vi "氨氮通讯.vi"() -> ()   [LabVIEW 2016, in "斯坦道氨氮.lvlib"]
uses:
  <vilib>/NI/Modbus Library/API/Wrapper/Create TCP Slave.vi
  <vilib>/Utility/config.llb/Write Key (String).vi
  <vilib>/Plasmionique/MB Master/MB_Master/MB_Master.lvclass
  <vilib>/NI/Modbus Library/API/slave/Modbus Slave.lvclass
  <vilib>/Utility/config.llb/NI_LVConfig.lvlib
  <vilib>/Plasmionique/MB Master/MB Master.lvlib
  <vilib>/NI/Modbus Library/API/Wrapper/API Main.lvlib
panel:
  out "测量数据区":T1 {"单位" items=["ug/L", "mg/L", "ppm", "mg/m3", "cm", "ppb", "ug/m3", "%", "nmol/mol", "umol/mol", "MPN/L", "MPN/100ml", "ng/m3", "NTU", "无量纲", "ms/cm", "us/cm", "℃", "mV", "万个/L"]}
  out "状态告警区":u16[](array[numeric])
  out "测量数据区":u16[](array[numeric])
  out "序列号":string
  out "状态告警区":T2
  out "status":bool
  out "关键参数区":T3
  in  "读关键参数区":bool
  in  "读状态告警区":bool
  in  "读测量数据区":bool
  in  "站号":u16(ring) items=["总磷"=1, "氨氮"=3]
  in  "停止":bool
  in  "启动":bool
  in  "控制命令":u16(ring) items=["启动测量"=1, "标样核查"=2, "零点核查"=3, "跨度核查"=4, "空白测试"=5, "平行样测试"=6, "加标回收"=7, "空白校准"=8, "标样校准"=9, "初始化（清洗）"=10, "停止测试"=11, "仪器重启"=12, "校时"=13, "模式设置"=14, "测量间隔设置"=15]
  in  "控制命令参数":u16[](array[numeric]) format="%04xH"
  in  "VISA Resource":refnum<visa-resource-name>
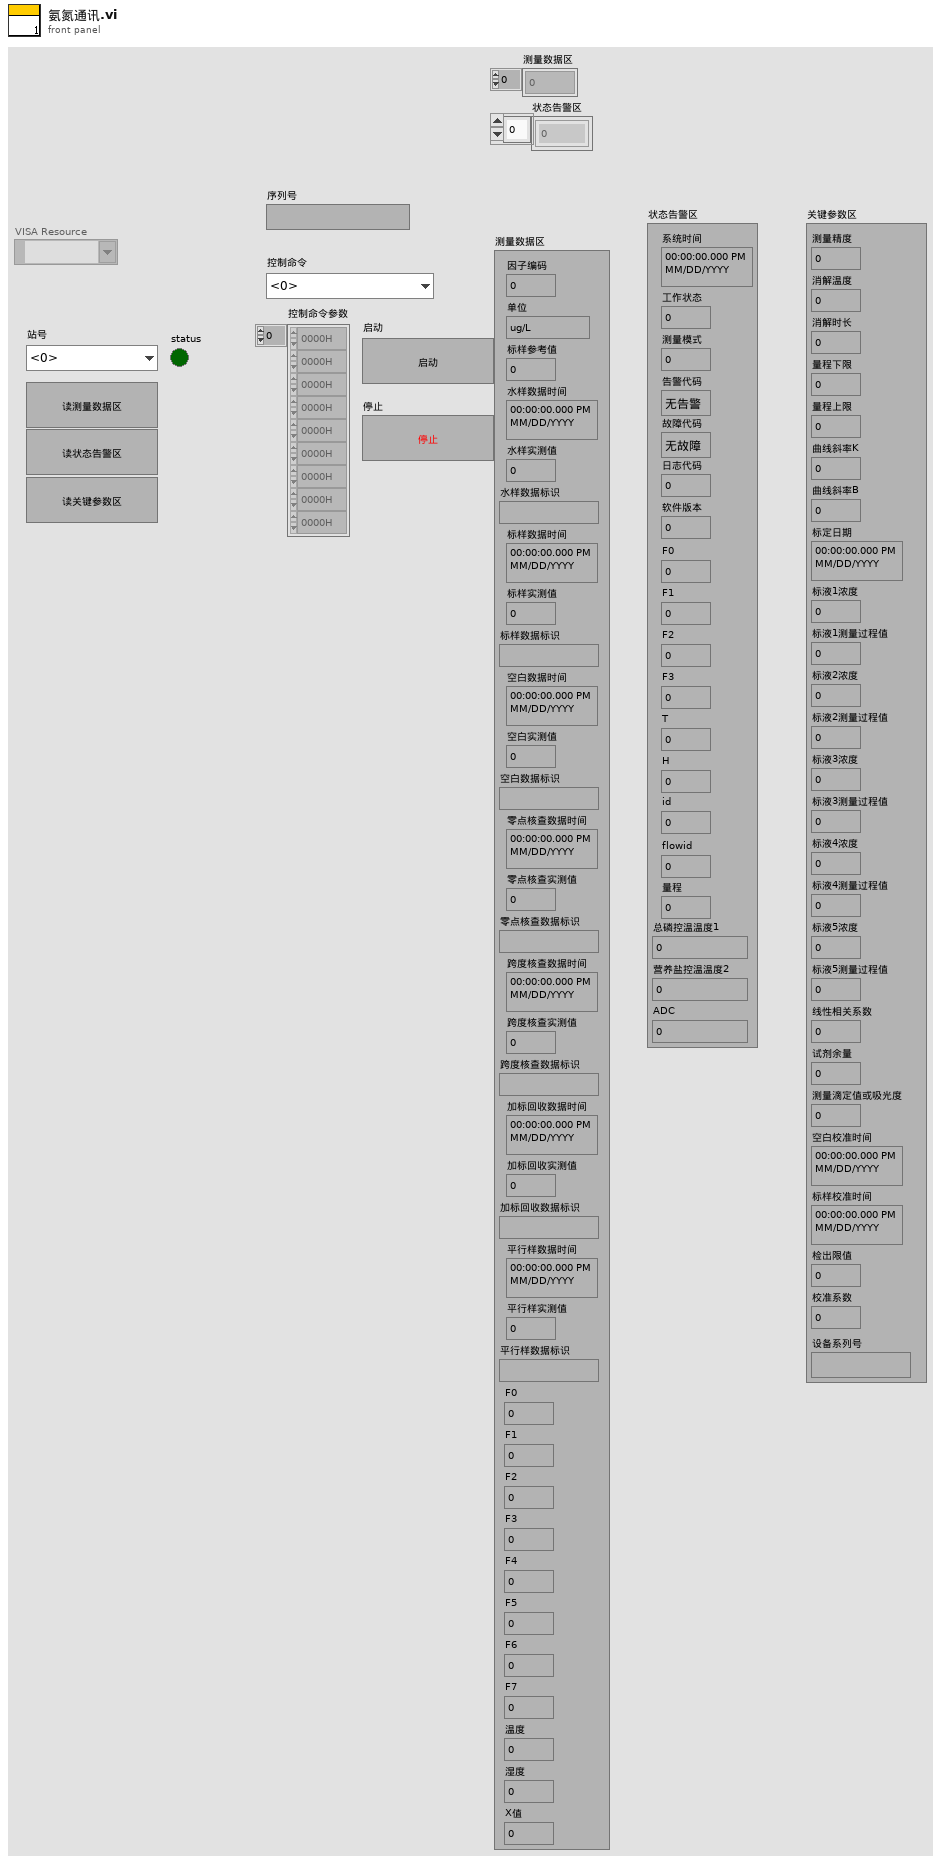
[diagram p1: front panel]
types:
  T1 = cluster{"因子编码":u32, "单位":u16, "标样参考值":sgl, "水样数据时间":timestamp, "水样实测值":sgl, "水样数据标识":string, "标样数据时间":timestamp, "标样实测值":sgl, "标样数据标识":string, "空白数据时间":timestamp, "空白实测值":sgl, "空白数据标识":string, "零点核查数据时间":timestamp, "零点核查实测值":sgl, "零点核查数据标识":string, "跨度核查数据时间":timestamp, "跨度核查实测值":sgl, "跨度核查数据标识":string, "加标回收数据时间":timestamp, "加标回收实测值":sgl, "加标回收数据标识":string, "平行样数据时间":timestamp, "平行样实测值":sgl, "平行样数据标识":string, "F0":sgl, "F1":sgl, "F2":sgl, "F3":sgl, "F4":sgl, "F5":sgl, "F6":sgl, "F7":sgl, "温度":sgl, "湿度":sgl, "X值":sgl}
  T2 = cluster{"系统时间":timestamp, "工作状态":u16, "测量模式":u16, "告警代码":enum16{"无告警", "缺试剂告警", "缺水样告警", "缺蒸馏水告警", "缺标液告警", "仪表漏液告警", "标定异常告警", "超量程告警", "加热异常", "低试剂预警", "超上限告警", "超下限告警", "仪表内部其他异常", "滴定异常告警", "电极异常告警", "量程切换告警", "参数设置告警", "PH电极电位异常", "电导率电极异常", "浊度光度异常", "溶解氧电极异常", "溶解氧光强异常", "温度异常告警", "PH异常告警", "溶解氧异常告警", "电导率异常告警", "浊度异常告警", "叶绿素异常告警", "藻密度异常告警", "蓝绿藻异常告警", "ORP异常告警", "氨氮异常告警", "清洁刷异常告警", "SD卡异常告警", "蓝牙异常告警", "Wifi异常告警", "流程异常告警"}, "故障代码":enum16{"无故障", "电机故障", "温度故障", "通讯故障", "滴定故障"}, "日志代码":u16, "软件版本":u16, "F0":sgl, "F1":sgl, "F2":sgl, "F3":sgl, "T":sgl, "H":sgl, "id":u16, "flowid":u16, "量程":u16, "ADC":sgl, "营养盐控温温度2":sgl, "总磷控温温度1":sgl}
  T3 = cluster{"测量精度":u16, "消解温度":u16, "消解时长":u16, "量程下限":sgl, "量程上限":sgl, "曲线斜率K":sgl, "曲线斜率B":sgl, "标定日期":timestamp, "标液1浓度":sgl, "标液1测量过程值":sgl, "标液2浓度":sgl, "标液2测量过程值":sgl, "标液3浓度":sgl, "标液3测量过程值":sgl, "标液4浓度":sgl, "标液4测量过程值":sgl, "标液5浓度":sgl, "标液5测量过程值":sgl, "线性相关系数":sgl, "试剂余量":u32, "测量滴定值或吸光度":sgl, "空白校准时间":timestamp, "标样校准时间":timestamp, "检出限值":sgl, "校准系数":sgl, "设备系列号":string}
  T4 = typedef "NI_LVConfig.lvlib/Config Data RefNum.ctl" = refnum<k1>
  T5 = enum8{"Enabled", "Disabled", "Disabled and Grayed Out"}
  T6 = cluster{"系统时间":timestamp, "工作状态":enum16{"空闲", "水样测试", "标样核查", "零点核查", "跨度核查", "空白测试", "平行样测试", "加标回收", "空白校准", "标样校准", "初始化（清洗）"}, "测量模式":enum16{"待机", "连续模式", "周期模式", "定点模式", "受控模式", "手动模式"}, "告警代码":enum16{"无告警", "缺试剂告警", "缺水样告警", "缺蒸馏水告警", "缺标液告警", "仪表漏液告警", "标定异常告警", "超量程告警", "加热异常", "低试剂预警", "超上限告警", "超下限告警", "仪表内部其他异常", "滴定异常告警", "电极异常告警", "量程切换告警", "参数设置告警", "PH电极电位异常", "电导率电极异常", "浊度光度异常", "溶解氧电极异常", "溶解氧光强异常", "温度异常告警", "PH异常告警", "溶解氧异常告警", "电导率异常告警", "浊度异常告警", "叶绿素异常告警", "藻密度异常告警", "蓝绿藻异常告警", "ORP异常告警", "氨氮异常告警", "清洁刷异常告警", "SD卡异常告警", "蓝牙异常告警", "Wifi异常告警", "流程异常告警"}, "故障代码":enum16{"无故障", "电机故障", "温度故障", "通讯故障", "滴定故障"}, "日志代码":u16, "软件版本":u16, "F0":sgl, "F1":sgl, "F2":sgl, "F3":sgl, "T":sgl, "H":sgl, "id":u16, "flowid":u16, "量程":u16, "总磷控温温度1":sgl, "营养盐控温温度2":sgl, "ADC":sgl}
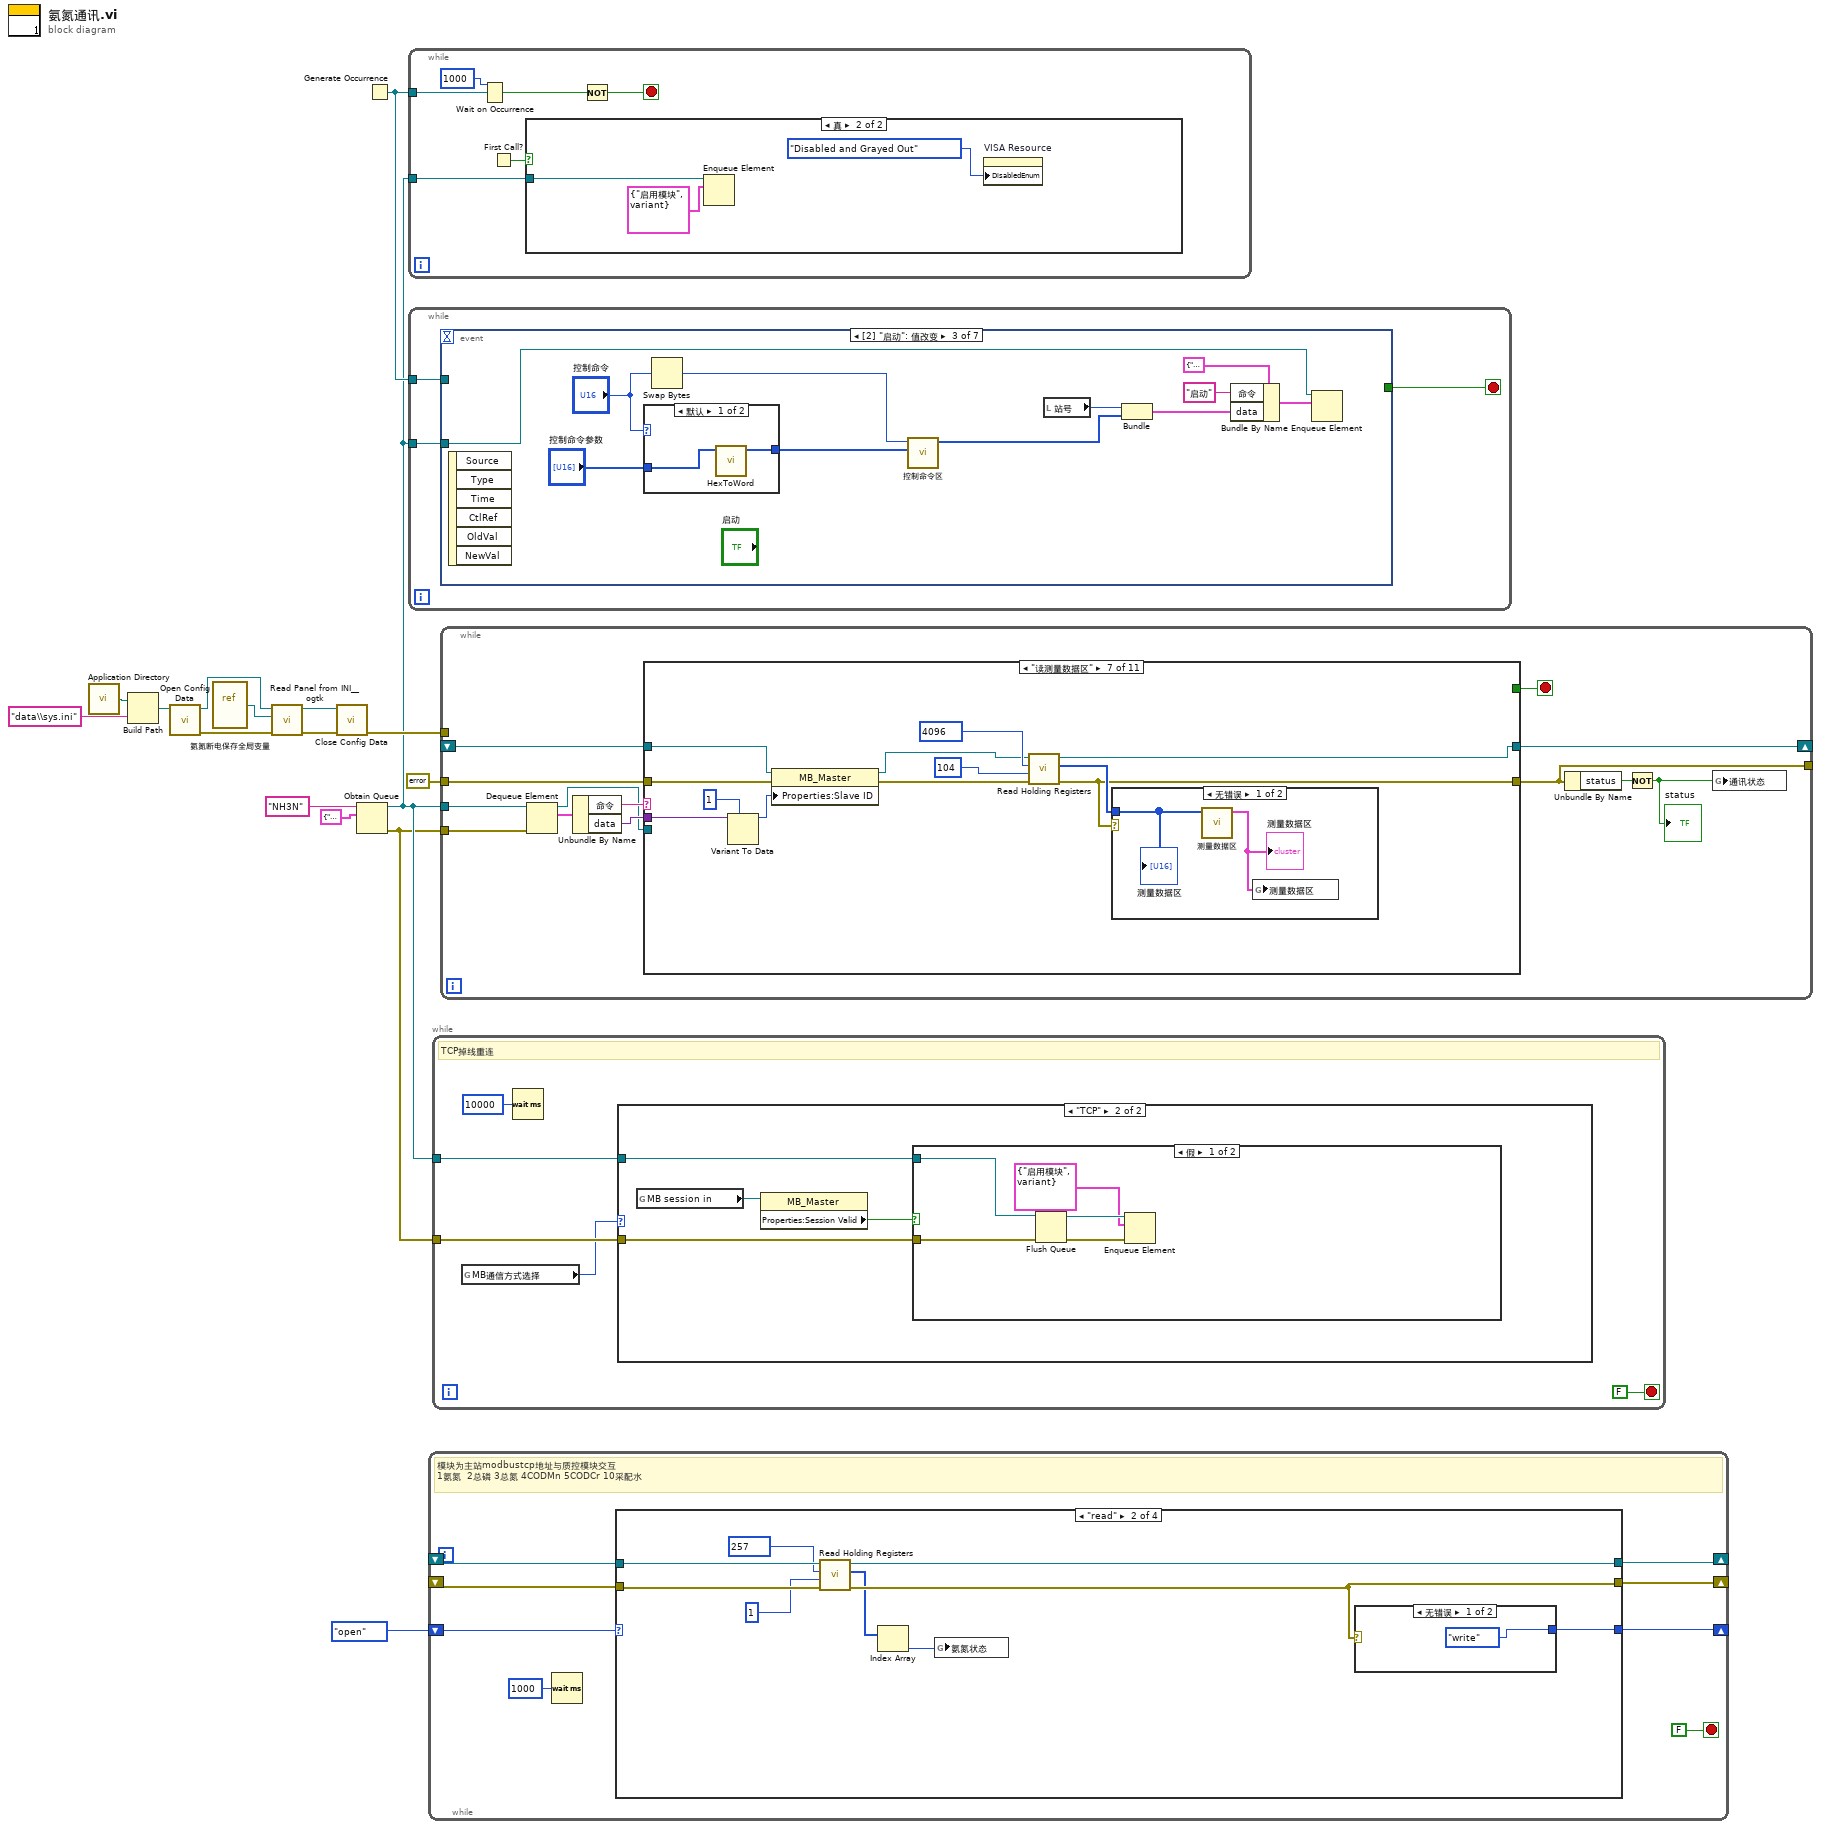
[diagram p0: block diagram]
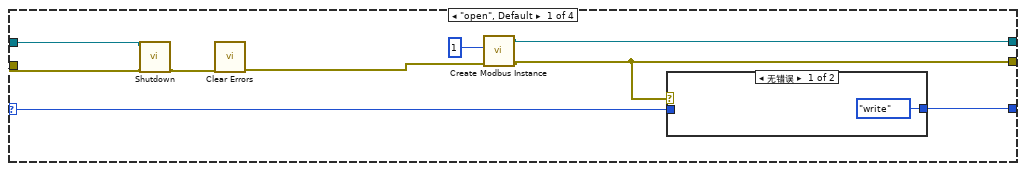
[diagram p4: hidden frame]
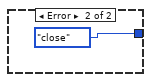
[diagram p6: hidden frame]
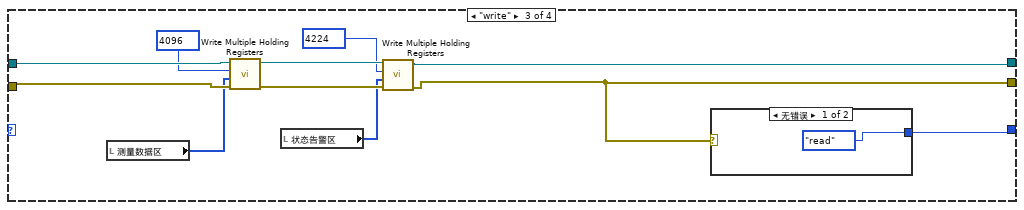
[diagram p7: hidden frame]
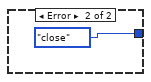
[diagram p8: hidden frame]
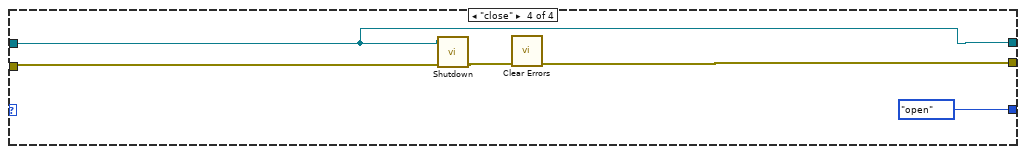
[diagram p9: hidden frame]
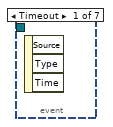
[diagram p11: hidden frame]
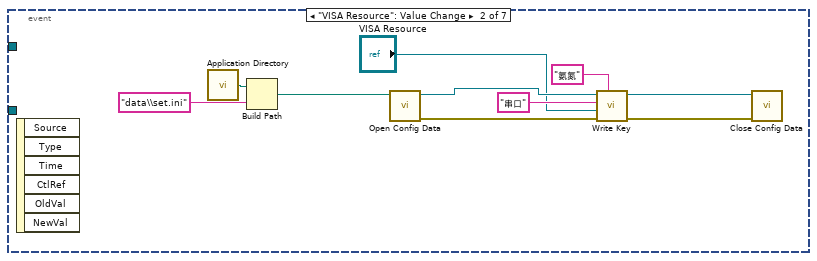
[diagram p12: hidden frame]
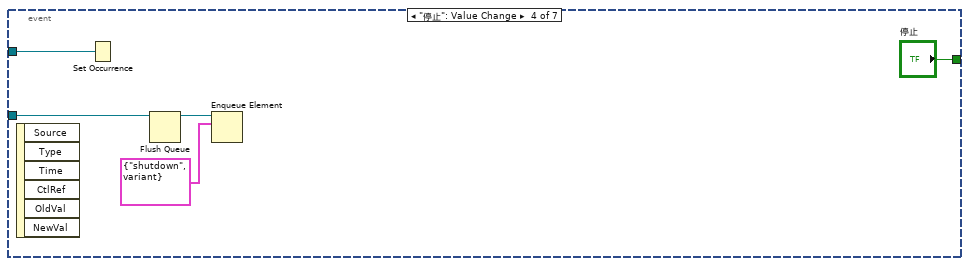
[diagram p14: hidden frame]
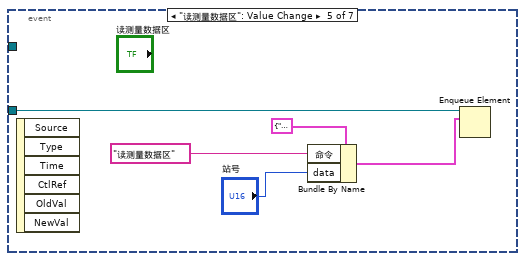
[diagram p15: hidden frame]
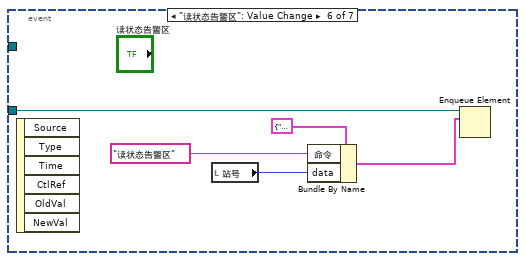
[diagram p16: hidden frame]
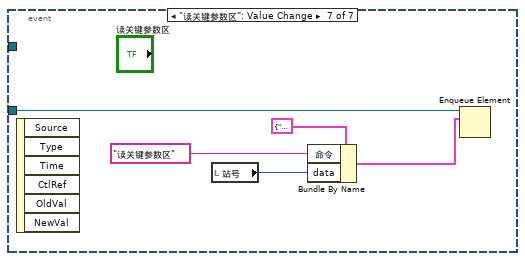
[diagram p17: hidden frame]
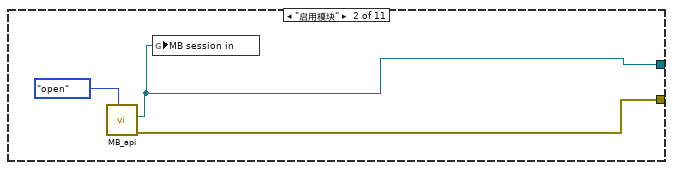
[diagram p19: hidden frame]
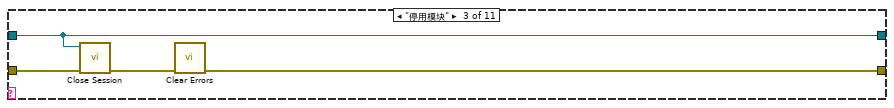
[diagram p20: hidden frame]
diagram:
  n1 = call <vilib>:"Application Directory.vi"() -> ("Application Directory"=w5:path)
  n2 = Build Path(base path=w5, name or relative path="data\\sys.ini" ("名称或相对路径")) -> (appended path=w7:path)
  n3 = call <vilib>:"Open Config Data.vi"("configuration file path"=w7) -> ("error out"=w11:errorcluster, "refnum"=w8:T4)  [unwired: 8 in, 1 out]
  n4 = vi-ref "氨氮断电保存全局变量.vi"() -> (w9:refnum<vi>)
  n5 = call <userlib>:"Read Panel from INI__ogtk.vi"("error in (no error)"=w11, "VI ref"=w9, "refnum"=w8) -> ("error out"=w12:errorcluster, "refnum out"=w10:T4)  [unwired: 7 in]
  n6 = call <vilib>:"Close Config Data.vi"("error in (no error)"=w12, "refnum"=w10) -> ("error out"=w4:errorcluster)  [unwired: 8 in, 1 out]
  n7 = Obtain Queue(name (unnamed)="NH3N" ("名称（未命名）"), element data type=cluster{"命令":string, "data":variant} {"命令"="", "data"=variant}) -> (queue out=w2:refnum<queue>, error out=w1:errorcluster)  [unwired: 3 in, 1 out]
  n8 = Generate Occurrence() -> (w13:refnum<k4>)
  n9 = while {
    tunnel: w13 -> [w22]
    tunnel: w2 -> [w18]
    stop <- w19 stop-if-true
    n10 = Wait on Occurrence(2:w22, 3:1000 ("毫秒超时(-1)")) -> (0:w20:bool)  [unwired: 1 in]
    n11 = First Call?() -> (First Call?: T/F=w17:bool)
    n12 = case shown="真" w17 {
      tunnel: w18 -> [_ w24]
      frame False {
      }
      frame True {
        n13 = Enqueue Element(queue=w24, element=cluster{"命令":string, "data":variant} {"命令"="启用模块", "data"=variant} ("元素")) -> ()  [unwired: 2 in, 3 out]
        n14 = property on="VISA Resource" class="VISAName"("DisabledEnum"=T5."Disabled and Grayed Out" ("禁用")) -> ()  [unwired: 2 in, 2 out]
      }
    }
    n15 = Not(x=w20) -> (.not. x?=w19:bool)
  }
  n16 = while {
    tunnel: w2 -> [w28]
    tunnel: w13 -> [w26]
    stop <- w27 stop-if-true
    n17 = event shown="[2] \"启动\": 值改变" {
      selector: _ -> [_ _ _ _ _ _ _]
      dyn-events: _ -> [_ _ _ _ _ _ _]
      timeout: _ -> [_ _ _ _ _ _ _]
      tunnel: w28 -> [_ _ w49 w56 w62 w67 w72]
      tunnel: [_ _ _ "停止" _ _ _] -> w27
      tunnel: w26 -> [_ _ _ w53 _ _ _]
      event Timeout {
        n18 = event-data() -> ()  [unwired: 1 in, 3 out]
      }
      event "VISA Resource": Value Change {
        n19 = event-data() -> ()  [unwired: 1 in, 6 out]
        n20 = call <vilib>:"Application Directory.vi"() -> ("Application Directory"=w31:path)
        n21 = Build Path(base path=w31, name or relative path="data\\set.ini" ("名称或相对路径")) -> (appended path=w32:path)
        n22 = call <vilib>:"Open Config Data.vi"("configuration file path"=w32) -> ("error out"=w38:errorcluster, "refnum"=w37:T4)  [unwired: 8 in, 1 out]
        n23 = call-poly <vilib>:"Write Key.vi"("section"="氨氮", "error in (no error)"=w38, "value"="VISA Resource", "key"="串口", "refnum"=w37) -> ("error out"=w34:errorcluster, "refnum out"=w30:T4)  [unwired: 4 in, 1 out]
        n24 = call <vilib>:"Close Config Data.vi"("error in (no error)"=w34, "refnum"=w30) -> ()  [unwired: 8 in, 2 out]
      }
      event "启动": Value Change {
        n25 = event-data() -> ()  [unwired: 1 in, 6 out]
        n26 = case shown="默认" "控制命令" {
          tunnel: "控制命令参数" -> [w51 w52]
          tunnel: [w50 w52] -> w39
          frame Default {
            n27 = call "HexToWord.vi"("数组"=w51) -> ("WORD"=w50:u16[])  [unwired: 10 in]
          }
          frame 13 {
          }
        }
        n28 = Swap Bytes(anything="控制命令") -> (byte swapped=w42:u16)
        n29 = call "控制命令区.vi"("控制命令参数"=w39, "控制命令"=w42) -> ("控制命令"=w45:u16[])  [unwired: 9 in]
        n30 = local read "站号"() -> (w44:u16)
        n31 = Bundle("站号"=w44, "控制命令"=w45) -> (w43:cluster{"站号":u16, "控制命令":u16[]})  [unwired: 1 in]
        n32 = Bundle By Name(cluster=cluster{"命令":string, "data":variant} {"命令"="", "data"=variant} ("元素"), "命令"="启动", "data"=w43) -> (w47:cluster{"命令":string, "data":variant})
        n33 = Enqueue Element(queue=w49, element=w47) -> ()  [unwired: 2 in, 3 out]
      }
      event "停止": Value Change {
        n34 = event-data() -> ()  [unwired: 1 in, 6 out]
        n35 = Set Occurrence(w53) -> ()
        n36 = Flush Queue(queue=w56) -> (queue out=w55:refnum<queue>)  [unwired: 1 in, 2 out]
        n37 = Enqueue Element(queue=w55, element=cluster{"命令":string, "data":variant} {"命令"="shutdown", "data"=variant} ("元素")) -> ()  [unwired: 2 in, 3 out]
      }
      event "读测量数据区": Value Change {
        n38 = event-data() -> ()  [unwired: 1 in, 6 out]
        n39 = Bundle By Name(cluster=cluster{"命令":string, "data":variant} {"命令"="", "data"=variant} ("元素"), "命令"="读测量数据区", "data"="站号") -> (w60:cluster{"命令":string, "data":variant})
        n40 = Enqueue Element(queue=w62, element=w60) -> ()  [unwired: 2 in, 3 out]
      }
      event "读状态告警区": Value Change {
        n41 = event-data() -> ()  [unwired: 1 in, 6 out]
        n42 = local read "站号"() -> (w63:u16)
        n43 = Bundle By Name(cluster=cluster{"命令":string, "data":variant} {"命令"="", "data"=variant} ("元素"), "命令"="读状态告警区", "data"=w63) -> (w65:cluster{"命令":string, "data":variant})
        n44 = Enqueue Element(queue=w67, element=w65) -> ()  [unwired: 2 in, 3 out]
      }
      event "读关键参数区": Value Change {
        n45 = event-data() -> ()  [unwired: 1 in, 6 out]
        n46 = local read "站号"() -> (w68:u16)
        n47 = Bundle By Name(cluster=cluster{"命令":string, "data":variant} {"命令"="", "data"=variant} ("元素"), "命令"="读关键参数区", "data"=w68) -> (w70:cluster{"命令":string, "data":variant})
        n48 = Enqueue Element(queue=w72, element=w70) -> ()  [unwired: 2 in, 3 out]
      }
    }
  }
  n49 = while {
    shift-right: [w78] -> _
    shift-left: _ -> [w80]
    shift-right: [w77] -> _
    shift-left: _ -> [w79]
    shift-right: [w74] -> _
    shift-left: enum16{"open", "read", "write", "close"}."open" -> [w75]
    stop <- FALSE stop-if-true
    # "模块为主站modbustcp地址与质控模块交互\n1氨氮  2总磷 3总氮 4CODMn 5CODCr 10采配水"
    n50 = Wait (ms)(milliseconds to wait=u32 1000 ("等待时间（毫秒）")) -> ()  [unwired: 1 out]
    n51 = case shown="\"read\"" w75 {
      selector: w75 -> [w89 _ _ _]
      tunnel: w80 -> [w83 w99 w112 w118]
      tunnel: w79 -> [w82 w97 w111 w117]
      tunnel: [w86 w98 w107 w118] -> w78
      tunnel: [w85 w96 w106 w120] -> w77
      tunnel: [w88 w100 w113 enum16{"open", "read", "write", "close"}."open"] -> w74
      frame "open", Default {
        n52 = call-dynamic "Shutdown.vi"("error in"=w82, "Modbus slave in"=w83) -> ("error out"=w81:errorcluster)  [unwired: 9 in]
        n53 = call <vilib>:"Clear Errors.vi"("error in (no error)"=w81) -> ("error out"=w84:errorcluster)  [unwired: 5 in, 1 out]
        n54 = call-poly <vilib>:"Create Modbus Instance.vi"("error in"=w84, "port (502)"=u16 1) -> ("error out"=w85:errorcluster, "TCP slave instance"=w86:refnum<class "Modbus Slave.lvclass">)  [unwired: 8 in]
        n55 = case shown="无错误" w85 {
          tunnel: w89 -> [_ w91]
          tunnel: [enum16{"open", "read", "write", "close"}."write" w91] -> w88
          frame No Error {
          }
          frame Error {
          }
        }
      }
      frame "read" {
        n56 = call-dynamic <vilib>:"Read Holding Registers.vi"("error in"=w97, "number of inputs"=u16 1, "starting address"=u16 257, "Modbus slave in"=w99) -> ("error out"=w96:errorcluster, "register values"=w93:u16[], "Modbus slave out"=w98:refnum<class "Modbus Slave.lvclass">)  [unwired: 5 in]
        n57 = Index Array(array=w93) -> (element=w92:u16)  [unwired: 1 in]
        n58 = global write "VAR氨氮全局变量.vi" "氨氮状态"(w92) -> ()
        n59 = case shown="无错误" w96 {
          tunnel: [enum16{"open", "read", "write", "close"}."write" enum16{"open", "read", "write", "close"}."close"] -> w100
          frame No Error {
          }
          frame Error {
          }
        }
      }
      frame "write" {
        n60 = local read "测量数据区"() -> (w105:u16[])
        n61 = call-dynamic "Write Multiple Holding Registers.vi"("error in"=w111, "registers to write"=w105, "starting address"=u16 4096, "Modbus slave in"=w112) -> ("error out"=w108:errorcluster, "Modbus slave out"=w109:refnum<class "Modbus Slave.lvclass">)  [unwired: 6 in]
        n62 = local read "状态告警区"() -> (w103:u16[])
        n63 = call-dynamic "Write Multiple Holding Registers.vi"("error in"=w108, "registers to write"=w103, "starting address"=u16 4224, "Modbus slave in"=w109) -> ("error out"=w106:errorcluster, "Modbus slave out"=w107:refnum<class "Modbus Slave.lvclass">)  [unwired: 6 in]
        n64 = case shown="无错误" w106 {
          tunnel: [enum16{"open", "read", "write", "close"}."read" enum16{"open", "read", "write", "close"}."close"] -> w113
          frame No Error {
          }
          frame Error {
          }
        }
      }
      frame "close" {
        n65 = call-dynamic "Shutdown.vi"("error in"=w117, "Modbus slave in"=w118) -> ("error out"=w116:errorcluster)  [unwired: 9 in]
        n66 = call <vilib>:"Clear Errors.vi"("error in (no error)"=w116) -> ("error out"=w120:errorcluster)  [unwired: 5 in, 1 out]
      }
    }
  }
  n67 = while "While循环" {
    tunnel: w2 -> [w123]
    tunnel: w1 -> [w122]
    stop <- FALSE stop-if-true
    # "TCP掉线重连"
    n68 = global read "氨氮断电保存全局变量.vi" "MB通信方式选择"() -> (w121:enum16{"串口", "TCP"})
    n69 = Wait (ms)(milliseconds to wait=u32 10000 ("等待时间（毫秒）")) -> ()  [unwired: 1 out]
    n70 = case shown="\"TCP\"" w121 {
      tunnel: w123 -> [_ w128]
      tunnel: w122 -> [_ w127]
      frame "串口", Default {
      }
      frame "TCP" {
        n71 = global read "VAR氨氮全局变量.vi" "MB session in"() -> (w126:refnum<class "MB_Master.lvclass">)
        n72 = property class="MB_Master"(reference=w126) -> ("Properties:Session Valid"=w129:bool)  [unwired: 1 in, 2 out]
        n73 = case shown="假" w129 {
          tunnel: w128 -> [w132 _]
          tunnel: w127 -> [w131 _]
          frame False {
            n74 = Flush Queue(queue=w132, error in (no error)=w131) -> (queue out=w134:refnum<queue>, error out=w133:errorcluster)  [unwired: 1 out]
            n75 = Enqueue Element(queue=w134, element=cluster{"命令":string, "data":variant} {"命令"="启用模块", "data"=variant} ("元素"), error in (no error)=w133) -> ()  [unwired: 1 in, 3 out]
          }
          frame True {
          }
        }
      }
    }
  }
  n76 = while {
    tunnel: w2 -> [w147]
    tunnel: w1 -> [w146]
    shift-right: [w144] -> _
    shift-left: _ -> [w143]
    tunnel: errorcluster {"status"=FALSE, "code"=0, "source"=""} ("error out") -> [w142]
    tunnel: [w137] -> _
    tunnel: w4 -> [_]
    stop <- w145 stop-if-true
    n77 = Dequeue Element(queue=w147, error in (no error)=w146) -> (queue out=w138:refnum<queue>, element=w140:cluster{"命令":string, "data":variant})  [unwired: 1 in, 2 out]
    n78 = Unbundle By Name(w140) -> ("命令"=w141:string, "data"=w139:variant)
    n79 = case shown="\"读测量数据区\"" w141 {
      tunnel: w139 -> [_ _ _ w166 w177 w194 w203 w213 w228 w242 _]
      tunnel: w138 -> [_ _ _ _ _ _ _ _ _ _ w255]
      tunnel: [_ _ _ _ _ _ _ _ _ _ TRUE] -> w145
      tunnel: [w148 w151 w153 w169 w180 w196 w208 w222 w235 w249 w251] -> w144
      tunnel: [w149 w150 w154 w168 w179 w195 w197 w223 w236 w250 w252] -> w137
      tunnel: w143 -> [w148 _ w153 w165 w176 w193 w202 w216 w231 w245 w251]
      tunnel: w142 -> [w149 _ w156 w162 w173 w190 w200 w217 w232 w246 w253]
      frame Default {
      }
      frame "启用模块" {
        n80 = call "MB_api.vi"("STEP"=enum16{"open", "read", "write", "close"}."open") -> ("error out"=w150:errorcluster, "MB session out"=w151:refnum<class "MB_Master.lvclass">)  [unwired: 8 in, 1 out]
        n81 = global write "VAR氨氮全局变量.vi" "MB session in"(w151) -> ()
      }
      frame "停用模块" {
        n82 = call-dynamic "Close Session.vi"("error in (no error)"=w156, "MB session in"=w153) -> ("error out"=w155:errorcluster)  [unwired: 9 in]
        n83 = call <vilib>:"Clear Errors.vi"("error in (no error)"=w155) -> ("error out"=w154:errorcluster)  [unwired: 5 in, 1 out]
      }
      frame "启动" {
        n84 = Variant To Data(type=cluster{"站号":u16, "控制命令":u16[]} {"站号"=0, "控制命令"=[]} ("输出簇"), Variant=w166) -> (data=w160:cluster{"站号":u16, "控制命令":u16[]})  [unwired: 1 in, 1 out]
        n85 = Unbundle By Name(w160) -> ("站号"=w159:u16, "控制命令"=w157:u16[])
        n86 = property class="MB_Master"(reference=w165, error in=w162, "Properties:Slave ID"=w159) -> (reference out=w164:refnum<class "MB_Master.lvclass">, error out=w163:errorcluster)
        n87 = Index Array(array=w157) -> (element=w158:u16)  [unwired: 1 in]
        n88 = global write "VAR氨氮全局变量.vi" "控制命令"(w158) -> ()
        n89 = call <vilib>:"Write Multiple Registers.vi"("error in (no error)"=w163, "values"=w157, "starting address"=u16 4608, "MB session in"=w164) -> ("error out"=w168:errorcluster, "MB session out"=w169:refnum<class "MB_Master.lvclass">)  [unwired: 6 in]
      }
      frame "盲样测试" {
        n90 = Variant To Data(type=0, Variant=w177) -> (data=w170:i32)  [unwired: 1 in, 1 out]
        n91 = property class="MB_Master"(reference=w176, error in=w173, "Properties:Slave ID"=w170) -> (reference out=w175:refnum<class "MB_Master.lvclass">, error out=w174:errorcluster)
        n92 = case shown="默认" w170 {
          tunnel: [u16[] [] ("values") u16[] [33539, 0] ("values") u16[] [23555, 0] ("values")] -> w172
          frame Default {
          }
          frame 1 {
            # "总磷盲样测试命令"
          }
          frame 3 {
            # "氨氮盲样测试"
          }
        }
        n93 = call <vilib>:"Write Multiple Registers.vi"("error in (no error)"=w174, "values"=w172, "starting address"=u16 24592, "MB session in"=w175) -> ("error out"=w179:errorcluster, "MB session out"=w180:refnum<class "MB_Master.lvclass">)  [unwired: 6 in]
      }
      frame "debug" {
        n94 = Variant To Data(type=cluster{"站号":u16, "控制命令":u16[]} {"站号"=0, "控制命令"=[]} ("输出簇"), Variant=w194) -> (data=w188:cluster{"站号":u16, "控制命令":u16[]})  [unwired: 1 in, 1 out]
        n95 = Unbundle By Name(w188) -> ("站号"=w187:u16, "控制命令"=w185:u16[])
        n96 = property class="MB_Master"(reference=w193, error in=w190, "Properties:Slave ID"=w187) -> (reference out=w192:refnum<class "MB_Master.lvclass">, error out=w191:errorcluster)
        n97 = Index Array(array=w185) -> (element=w186:u16)  [unwired: 1 in]
        n98 = global write "VAR氨氮全局变量.vi" "控制命令"(w186) -> ()
        n99 = call <vilib>:"Write Multiple Registers.vi"("error in (no error)"=w191, "values"=w185, "starting address"=u16 24594, "MB session in"=w192) -> ("error out"=w195:errorcluster, "MB session out"=w196:refnum<class "MB_Master.lvclass">)  [unwired: 6 in]
      }
      frame "读测量数据区" {
        n100 = Variant To Data(type=u8 1 ("Slave ID"), Variant=w203) -> (data=w204:u8)  [unwired: 1 in, 1 out]
        n101 = property class="MB_Master"(reference=w202, error in=w200, "Properties:Slave ID"=w204) -> (reference out=w201:refnum<class "MB_Master.lvclass">, error out=w199:errorcluster)
        n102 = call <vilib>:"Read Holding Registers.vi"("error in (no error)"=w199, "quantity"=u16 104, "starting address"=u16 4096, "MB session in"=w201) -> ("error out"=w197:errorcluster, "Registers"=w198:u16[], "MB session out"=w208:refnum<class "MB_Master.lvclass">)  [unwired: 5 in]
        n103 = case shown="无错误" w197 {
          tunnel: w198 -> [w210 _]
          frame No Error {
            n104 = call "测量数据区.vi"("数组"=w210) -> ("测量数据区"=w209:T1)  [unwired: 10 in]
            "测量数据区" <- w209
            n105 = global write "VAR氨氮全局变量.vi" "测量数据区"(w209) -> ()
            "测量数据区" <- w210
          }
          frame Error {
          }
        }
      }
      frame "读状态告警区" {
        n106 = Variant To Data(type=u8 1 ("Slave ID"), Variant=w213) -> (data=w218:u8)  [unwired: 1 in, 1 out]
        n107 = property class="MB_Master"(reference=w216, error in=w217, "Properties:Slave ID"=w218) -> (reference out=w215:refnum<class "MB_Master.lvclass">, error out=w214:errorcluster)
        n108 = call <vilib>:"Read Holding Registers.vi"("error in (no error)"=w214, "quantity"=u16 24, "starting address"=u16 4224, "MB session in"=w215) -> ("error out"=w223:errorcluster, "Registers"=w212:u16[], "MB session out"=w222:refnum<class "MB_Master.lvclass">)  [unwired: 5 in]
        "状态告警区" <- w212
        n109 = call "状态告警区.vi"("数组"=w212) -> ("状态告警区"=w211:T6)  [unwired: 10 in]
        "状态告警区" <- w211
        n110 = global write "VAR氨氮全局变量.vi" "状态告警区"(w211) -> ()
      }
      frame "读关键参数区" {
        n111 = Variant To Data(type=u8 1 ("Slave ID"), Variant=w228) -> (data=w226:u8)  [unwired: 1 in, 1 out]
        n112 = property class="MB_Master"(reference=w231, error in=w232, "Properties:Slave ID"=w226) -> (reference out=w230:refnum<class "MB_Master.lvclass">, error out=w229:errorcluster)
        n113 = call <vilib>:"Read Holding Registers.vi"("error in (no error)"=w229, "quantity"=u16 19, "starting address"=u16 4256, "MB session in"=w230) -> ("error out"=w236:errorcluster, "Registers"=w225:u16[], "MB session out"=w235:refnum<class "MB_Master.lvclass">)  [unwired: 5 in]
        n114 = call "关键参数区.vi"("数组"=w225) -> ("关键参数区"=w224:T3)  [unwired: 10 in]
        "关键参数区" <- w224
        n115 = global write "VAR氨氮全局变量.vi" "关键参数区"(w224) -> ()
      }
      frame "读序列号" {
        n116 = Variant To Data(type=u8 1 ("Slave ID"), Variant=w242) -> (data=w240:u8)  [unwired: 1 in, 1 out]
        n117 = property class="MB_Master"(reference=w245, error in=w246, "Properties:Slave ID"=w240) -> (reference out=w244:refnum<class "MB_Master.lvclass">, error out=w243:errorcluster)
        n118 = call <vilib>:"Read Holding Registers.vi"("error in (no error)"=w243, "quantity"=u16 6, "starting address"=u16 3, "MB session in"=w244) -> ("error out"=w250:errorcluster, "Registers"=w239:u16[], "MB session out"=w249:refnum<class "MB_Master.lvclass">)  [unwired: 5 in]
        n119 = call "HexToString.vi"("数组"=w239) -> ("STRING"=w238:string[])  [unwired: 10 in]
        n120 = Index Array(array=w238) -> (element=w237:string)  [unwired: 1 in]
        "序列号" <- w237
        n121 = global write "VAR氨氮全局变量.vi" "序列号"(w237) -> ()
      }
      frame "shutdown" {
        n122 = call-dynamic "Close Session.vi"("error in (no error)"=w253, "MB session in"=w251) -> ("error out"=w252:errorcluster)  [unwired: 9 in]
        n123 = Flush Queue(queue=w255) -> (queue out=w254:refnum<queue>)  [unwired: 1 in, 2 out]
        n124 = Release Queue(queue=w254) -> ()  [unwired: 2 in, 3 out]
      }
    }
    n125 = Unbundle By Name(w137) -> ("status"=w136:bool)
    n126 = Not(x=w136) -> (.not. x?=w135:bool)
    "status" <- w135
    n127 = global write "VAR氨氮全局变量.vi" "通讯状态"(w135) -> ()
  }
